vi "Init Switch.vi"(8 "error in (no error)":errorcluster, 11 "resource name":refnum<k15>) -> (0 "error out":errorcluster, 3 "instrument handle out":refnum<k15>)   [LabVIEW 2015]
uses:
  <instrlib>/niSwitch/niSwitch.llb/niSwitch Topologies.ctl
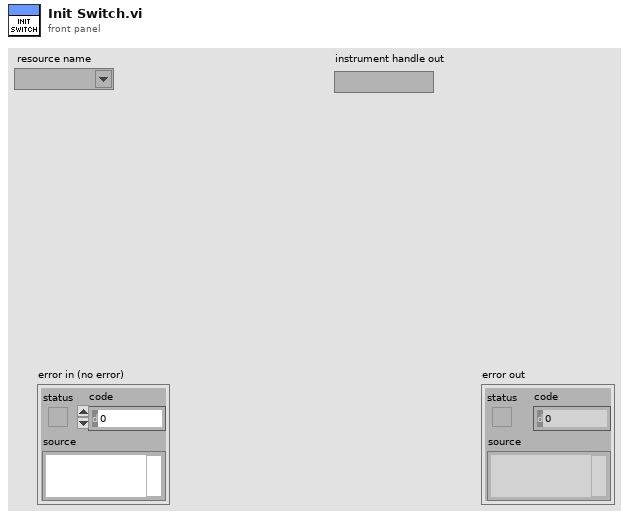
[diagram p1: front panel]
types:
  T1 = typedef "niSwitch Topologies.ctl" = string
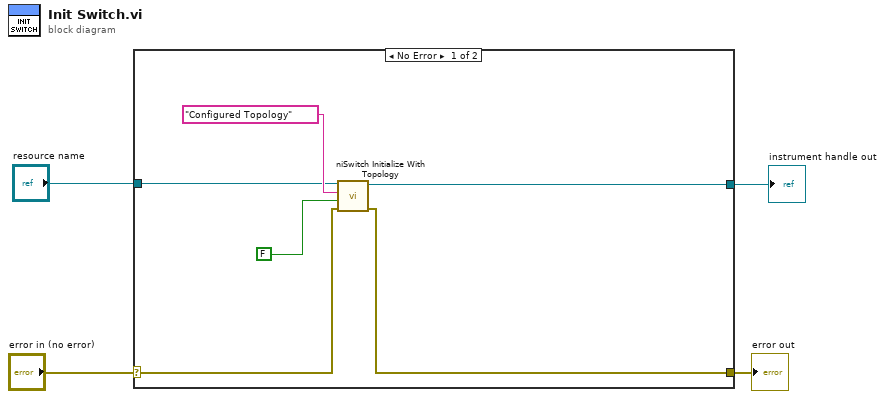
[diagram p0: block diagram]
diagram:
  n1 = case shown="No Error" "error in (no error)" {
    selector: "error in (no error)" -> [w8 w11]
    tunnel: [w9 w11] -> w3
    tunnel: "resource name" -> [w6 _]
    tunnel: [w5 _] -> w1
    frame No Error {
      n2 = call <instrlib>:"niSwitch Initialize With Topology.vi"("error in (no error)"=w8, "reset device (boolean value)"=FALSE, "topology name"=T1 "Configured Topology", "resource name"=w6) -> ("error out"=w9:errorcluster, "instrument handle out"=w5:refnum<k15>)  [unwired: 6 in]
    }
    frame Error {
    }
  }
  "error out" <- w3
  "instrument handle out" <- w1
